vi "S&E Annotation String.vi"(2 "Elevated priority":bool, 7 "Content":variant, 9 "error in":errorcluster) -> (8 "format string":string, 10 "error out":errorcluster)   [LabVIEW 2011]
uses:
  reate/S&E Anotationtype.ctl
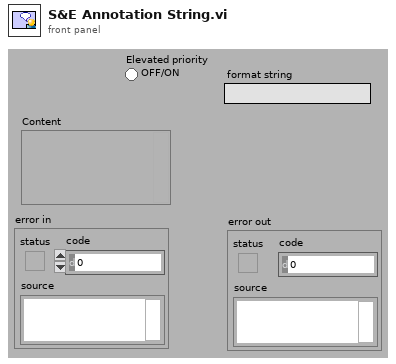
[diagram p1: front panel]
types:
  T1 = typedef "S&E Anotationtype.ctl" = cluster{"User":string, "Annotation":string}
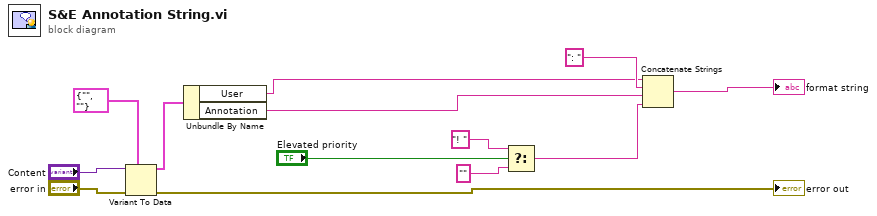
[diagram p0: block diagram]
diagram:
  n1 = Variant To Data(error in="error in", type=T1 {"User"="", "Annotation"=""} ("S&E Alarm"), Variant="Content") -> (data=w8:T1, error out=→"error out":errorcluster)
  n2 = Unbundle By Name(w8) -> ("User"=w5:string, "Annotation"=w10:string)
  n3 = Select(t="! " ("string"), s="Elevated priority", f="") -> (s? t:f=w1:string)
  n4 = Concatenate Strings(w5, ": " ("string"), w10, w1) -> (→"format string":string)
